vi "FGV_ConnectionStatus.vi"(4 "Enum":enum16{"Set", "LastContact", "Get"}(ring)) -> (5 "Seconds since last communication with MIDAS":dbl, 6 "MIDAS Connection OK":bool)   [LabVIEW 2018, in "feGEM DataPacker.lvlib"]
uses:
  feGEM DataPacker.lvlib
panel:
  out "Last Contact Time":timestamp
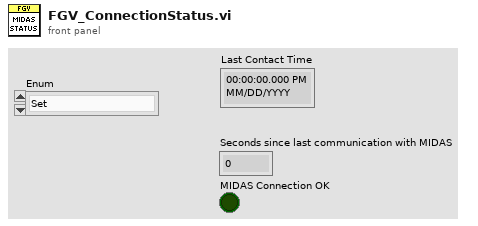
[diagram p1: front panel]
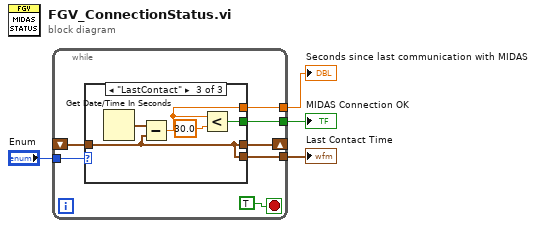
[diagram p0: block diagram]
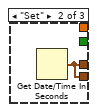
[diagram p3: hidden frame]
diagram:
  n1 = while {
    tunnel: "Enum" -> [w11]
    tunnel: [w8] -> w3
    shift-right: [w9] -> _
    shift-left: _ -> [w7]
    tunnel: [w6] -> w2
    tunnel: [w5] -> w1
    stop <- TRUE stop-if-true
    n2 = case shown="\"LastContact\"" w11 {
      tunnel: [w12 w13 w18] -> w9
      tunnel: [w12 w13 w18] -> w8
      tunnel: w7 -> [w12 _ w18]
      tunnel: [_ _ w16] -> w6
      tunnel: [_ _ w14] -> w5
      frame "Get", Default {
      }
      frame "Set" {
        n3 = Get Date/Time In Seconds() -> (seconds since 1Jan1904=w13:timestamp)
      }
      frame "LastContact" {
        n4 = Get Date/Time In Seconds() -> (seconds since 1Jan1904=w17:timestamp)
        n5 = Subtract(x=w17, y=w18) -> (x-y=w16:dbl)
        n6 = Less?(x=w16, y=30.0) -> (x < y?=w14:bool)
      }
    }
  }
  "Last Contact Time" <- w3
  "Seconds since last communication with MIDAS" <- w2
  "MIDAS Connection OK" <- w1
